vi "complete standard cycle shift.vi"(7 "read write shift":string(combo), 8 "error in":errorcluster, 11 "DATA CLUSTER in":T1) -> (0 "error out":errorcluster, 3 "DATA CLUSTER out":T1)   [LabVIEW 2016]
doc: "Shift register used to transport data from one analysis vi to another"
uses:
  controls/data control cluster.ctl
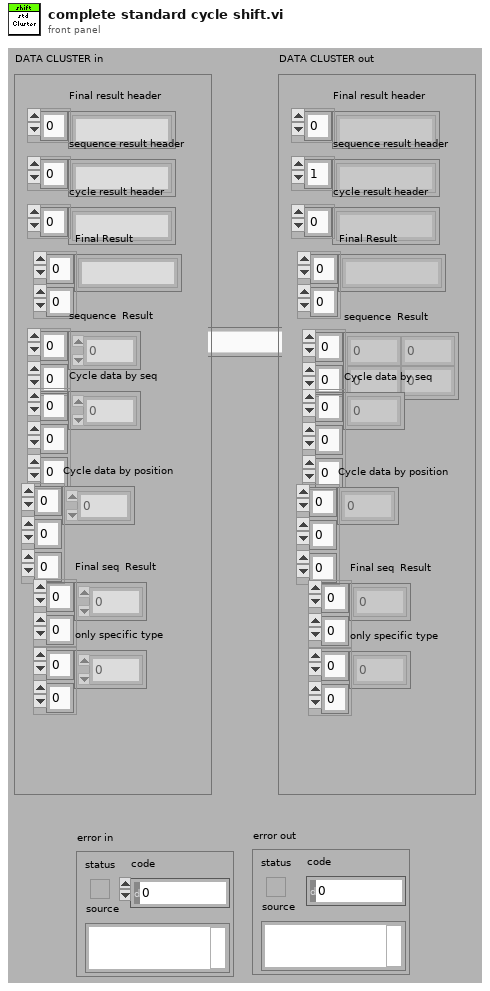
[diagram p1: front panel]
types:
  T1 = typedef "data control cluster.ctl" = cluster{"Final result header":string[], "sequence result header":string[], "cycle result header ":string[], "Final Result":string[][], "sequence  Result":dbl[][], "Cycle data by seq":dbl[][][], "Cycle data by position":dbl[][][], "Final seq  Result":dbl[][], "only specific type":dbl[][]}
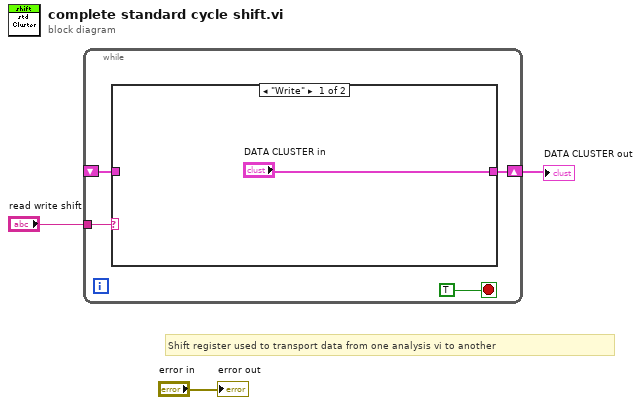
[diagram p0: block diagram]
diagram:
  # "Shift register used to transport data from one analysis vi to another"
  n1 = while {
    tunnel: "read write shift" -> [w7]
    shift-right: [w6] -> w1
    shift-left: _ -> [w4]
    stop <- TRUE stop-if-true
    n2 = case shown="\"Write\"" w7 {
      tunnel: ["DATA CLUSTER in" w9] -> w6
      tunnel: w4 -> [_ w9]
      frame "Write" {
      }
      frame "Read", Default {
      }
    }
  }
  "DATA CLUSTER out" <- w1
  "error out" <- "error in"
